vi "Boolean(0,1).vi"() -> ()   [LabVIEW 2021]
panel:
  out "0, 1":i16
  out "Boolean 2":bool
  in  "Boolean":bool
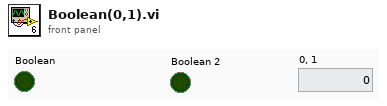
[diagram p1: front panel]
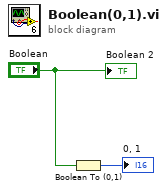
[diagram p0: block diagram]
diagram:
  n1 = Boolean To (0,1)(Boolean="Boolean") -> (0, 1=→"0, 1":i16)
  "Boolean 2" <- "Boolean"
